vi "settings UL array.vi"(9 "Settings UL":dbl[](array[numeric]), 11 "Settings UL":T1 {"RPM" items=["TESTO", "TORSIOMETRO", "OTTICA"]; "PRESSIONE MANDATA" items=["P1", "P2", "P3"]; "PRESSIONE ASPIRAZIONE" items=["P1", "P2", "P3"]; "PORTATA SECONDARIA" items=["Q1", "Q2", "Q3"]; "PORTATA PRINCIPALE" items=["Q1", "Q2", "Q3"]; "T"."Medie" min=1 step=1; "Tq"."Medie" min=1 step=1; "N"."Medie" min=1 step=1; "P3"."Medie" min=1 step=1; "P2"."Medie" min=1 step=1; "P1"."Medie" min=1 step=1; "Q3"."Medie" min=1 step=1; "Q2"."Medie" min=1 step=1; "Q1"."Medie" min=1 step=1}) -> (1 "Settings UL out":T1 {"RPM" items=["TESTO", "TORSIOMETRO", "OTTICA"]; "PRESSIONE MANDATA" items=["P1", "P2", "P3"]; "PRESSIONE ASPIRAZIONE" items=["P1", "P2", "P3"]; "PORTATA SECONDARIA" items=["Q1", "Q2", "Q3"]; "PORTATA PRINCIPALE" items=["Q1", "Q2", "Q3"]; "T"."Medie" min=1 step=1; "Tq"."Medie" min=1 step=1; "N"."Medie" min=1 step=1; "P3"."Medie" min=1 step=1; "P2"."Medie" min=1 step=1; "P1"."Medie" min=1 step=1; "Q3"."Medie" min=1 step=1; "Q2"."Medie" min=1 step=1; "Q1"."Medie" min=1 step=1}, 3 "Settings UL out":dbl[](array[numeric]))   [LabVIEW 2019]
uses:
  TypeDef/cDAQ Settings UL.ctl
  TypeDef/SETUP INGRESSO.ctl
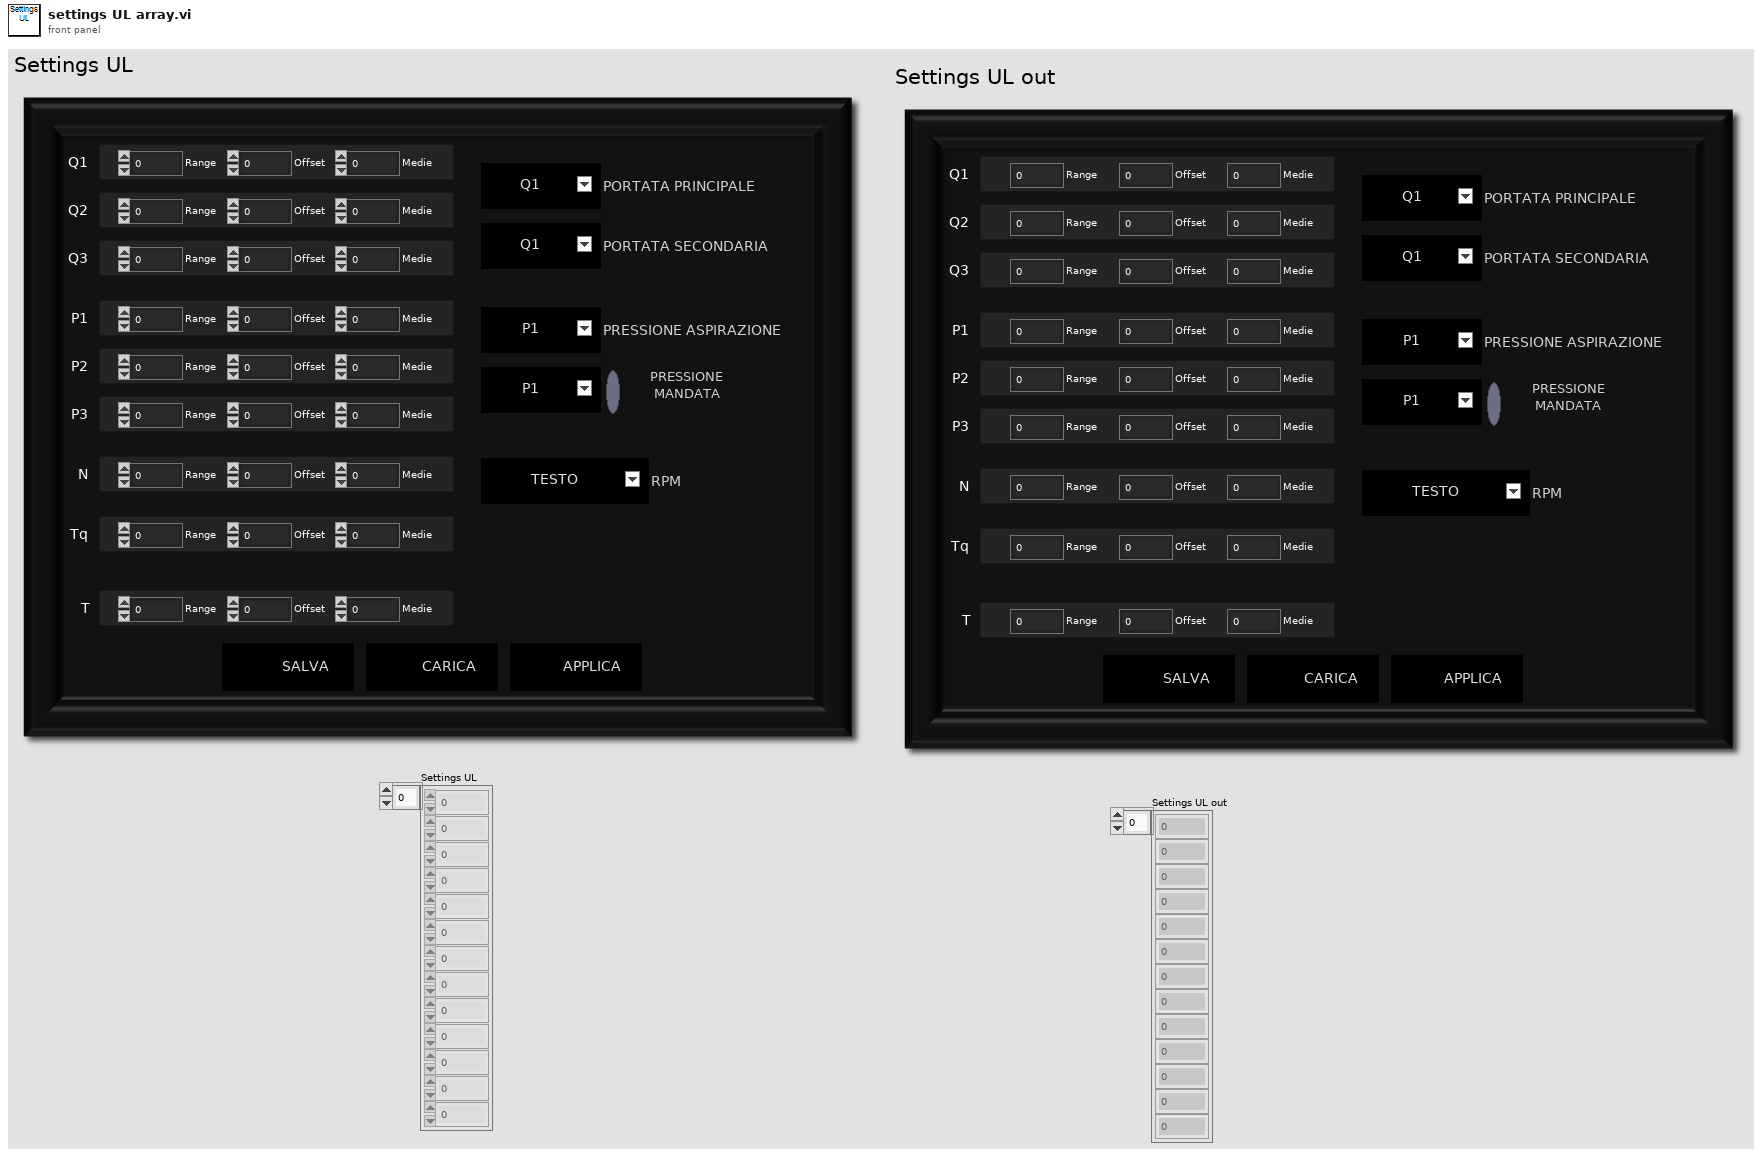
[diagram p1: front panel]
types:
  T1 = typedef "cDAQ Settings UL.ctl" = cluster{"SALVA":bool, "CARICA":bool, "APPLICA":bool, "Q1":T2, "Q2":T2, "Q3":T2, "P1":T2, "P2":T2, "P3":T2, "N":T2, "Tq":T2, "T":T2, "PORTATA PRINCIPALE":u16, "PORTATA SECONDARIA":u16, "PRESSIONE ASPIRAZIONE":u16, "PRESSIONE MANDATA":u16, "RPM":u16, "differenziale?":bool}
  T2 = typedef "SETUP INGRESSO.ctl" = cluster{"Range":dbl, "Offset":dbl, "Medie":u8}
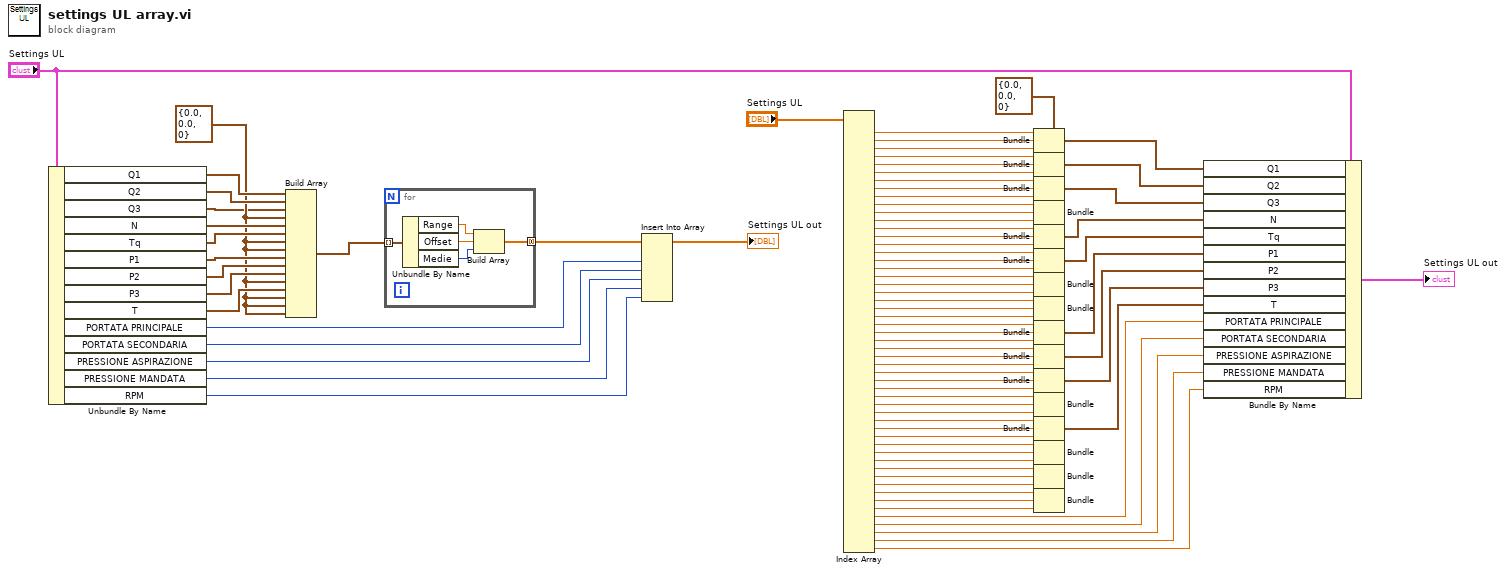
[diagram p0: block diagram]
diagram:
  w35 = T2 {"Range"=0.0, "Offset"=0.0, "Medie"=0} ("element")
  w27 = T2 {"Range"=0.0, "Offset"=0.0, "Medie"=0} ("Q1")
  n1 = Unbundle By Name("Settings UL") -> ("Q1"=w43:T2, "Q2"=w42:T2, "Q3"=w34:T2, "N"=w41:T2, "Tq"=w40:T2, "P1"=w39:T2, "P2"=w38:T2, "P3"=w37:T2, "T"=w36:T2, "PORTATA PRINCIPALE"=w49:u16, "PORTATA SECONDARIA"=w48:u16, "PRESSIONE ASPIRAZIONE"=w47:u16, "PRESSIONE MANDATA"=w46:u16, "RPM"=w45:u16)
  n2 = Build Array(w43, w42, w34, w35, w41, w40, w35, w35, w39, w38, w37, w35, w36, w35, w35, w35) -> (w82:T2[])
  n3 = for {
    tunnel: w82 -> [w89] mode=indexing
    tunnel: [w85] -> w50 mode=concatenating
    n4 = Unbundle By Name(w89) -> ("Range"=w88:dbl, "Offset"=w87:dbl, "Medie"=w86:u8)
    n5 = Build Array(w88, w87, w86) -> (w85:dbl[])
  }
  n6 = Insert Into Array(array=w50, new element #1=w49, new element #2=w48, new element #3=w47, new element #4=w46, new element #5=w45) -> (→"Settings UL out":dbl[])  [unwired: 1 in]
  n7 = Index Array(array="Settings UL") -> (element #1=w80:dbl, element #2=w79:dbl, element #3=w78:dbl, element #4=w77:dbl, element #5=w76:dbl, element #6=w75:dbl, element #7=w74:dbl, element #8=w73:dbl, element #9=w72:dbl, element #10=w71:dbl, element #11=w70:dbl, element #12=w69:dbl, element #13=w68:dbl, element #14=w67:dbl, element #15=w66:dbl, element #16=w65:dbl, element #17=w64:dbl, element #18=w63:dbl, element #19=w62:dbl, element #20=w61:dbl, element #21=w60:dbl, element #22=w59:dbl, element #23=w58:dbl, element #24=w57:dbl, element #25=w56:dbl, element #26=w55:dbl, element #27=w54:dbl, element #28=w26:dbl, element #29=w25:dbl, element #30=w24:dbl, element #31=w23:dbl, element #32=w22:dbl, element #33=w21:dbl, element #34=w20:dbl, element #35=w19:dbl, element #36=w18:dbl, element #37=w17:dbl, element #38=w16:dbl, element #39=w15:dbl, element #40=w14:dbl, element #41=w13:dbl, element #42=w12:dbl, element #43=w11:dbl, element #44=w10:dbl, element #45=w9:dbl, element #46=w8:dbl, element #47=w7:dbl, element #48=w6:dbl, element #49=w5:dbl, element #50=w4:dbl, element #51=w3:dbl, element #52=w2:dbl, element #53=w1:dbl)  [unwired: 53 in]
  n8 = Bundle(cluster=w27, "Range"=w80, "Offset"=w79, "Medie"=w78) -> (w53:T2)
  n9 = Bundle(cluster=w27, "Range"=w77, "Offset"=w76, "Medie"=w75) -> (w52:T2)
  n10 = Bundle(cluster=w27, "Range"=w74, "Offset"=w73, "Medie"=w72) -> (w51:T2)
  n11 = Bundle(cluster=w27, "Range"=w71, "Offset"=w70, "Medie"=w69) -> ()  [unwired: 1 out]
  n12 = Bundle(cluster=w27, "Range"=w68, "Offset"=w67, "Medie"=w66) -> (w33:T2)
  n13 = Bundle(cluster=w27, "Range"=w65, "Offset"=w64, "Medie"=w63) -> (w32:T2)
  n14 = Bundle(cluster=w27, "Range"=w62, "Offset"=w61, "Medie"=w60) -> ()  [unwired: 1 out]
  n15 = Bundle(cluster=w27, "Range"=w59, "Offset"=w58, "Medie"=w57) -> ()  [unwired: 1 out]
  n16 = Bundle(cluster=w27, "Range"=w56, "Offset"=w55, "Medie"=w54) -> (w31:T2)
  n17 = Bundle(cluster=w27, "Range"=w26, "Offset"=w25, "Medie"=w24) -> (w30:T2)
  n18 = Bundle(cluster=w27, "Range"=w23, "Offset"=w22, "Medie"=w21) -> (w29:T2)
  n19 = Bundle(cluster=w27, "Range"=w20, "Offset"=w19, "Medie"=w18) -> ()  [unwired: 1 out]
  n20 = Bundle(cluster=w27, "Range"=w17, "Offset"=w16, "Medie"=w15) -> (w28:T2)
  n21 = Bundle(cluster=w27, "Range"=w14, "Offset"=w13, "Medie"=w12) -> ()  [unwired: 1 out]
  n22 = Bundle(cluster=w27, "Range"=w11, "Offset"=w10, "Medie"=w9) -> ()  [unwired: 1 out]
  n23 = Bundle(cluster=w27, "Range"=w8, "Offset"=w7, "Medie"=w6) -> ()  [unwired: 1 out]
  n24 = Bundle By Name(cluster="Settings UL", "Q1"=w53, "Q2"=w52, "Q3"=w51, "N"=w33, "Tq"=w32, "P1"=w31, "P2"=w30, "P3"=w29, "T"=w28, "PORTATA PRINCIPALE"=w5, "PORTATA SECONDARIA"=w4, "PRESSIONE ASPIRAZIONE"=w3, "PRESSIONE MANDATA"=w2, "RPM"=w1) -> (→"Settings UL out":T1)
